vi "请求注销.vi"(8 "error in (no error)":errorcluster caption="错误输入（无错误）", 10 "数据采集.lvclass":refnum<class "数据采集.lvclass">, 11 "数据存储 输入":refnum<class "数据存储.lvclass"> caption="DNL_LabVIEW Object in") -> (0 "error out":errorcluster caption="错误输出", 2 "数据采集.lvclass":refnum<class "数据采集.lvclass">, 3 "数据存储 输出":refnum<class "数据存储.lvclass"> caption="DNL_LabVIEW Object out")   [LabVIEW 2013, in "数据存储.lvclass"]
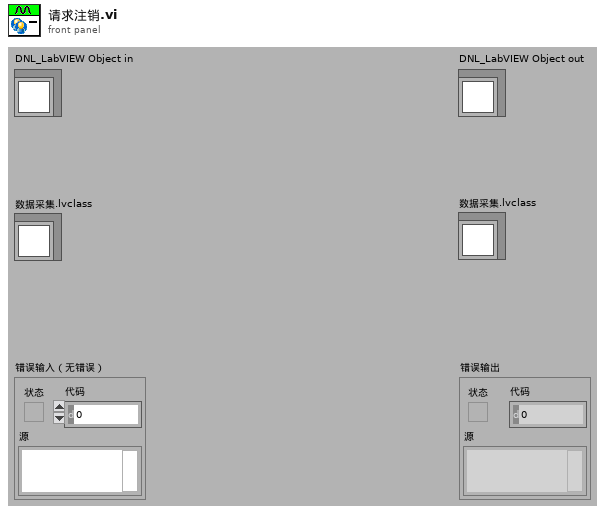
[diagram p1: front panel]
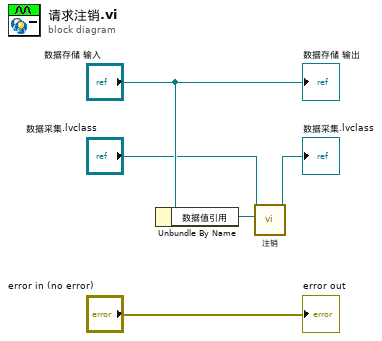
[diagram p0: block diagram]
diagram:
  n1 = Unbundle By Name("数据存储 输入") -> ("数据值引用"=w3:refnum<data-value>)
  n2 = call-dynamic "注销.vi"("数据值引用"=w3, "数据采集 输入"="数据采集.lvclass") -> ("数据采集 输出"=→"数据采集.lvclass":refnum<class "数据采集.lvclass">)  [unwired: 8 in, 1 out]
  "error out" <- "error in (no error)"
  "数据存储 输出" <- "数据存储 输入"
